vi "STM32.ADC.vi"(5 "Error":dbl, 6 "SampleRate":dbl=250000.0, 7 "Rate":dbl=1.0, 8 "Error In":errorcluster caption="错误输入", 9 "Points(X*4k)":u8=1 min=1 max=100, 10 "Channel":enum16{"Channel A", "Channel B"}(ring), 11 "VISA资源输入":refnum<visa-resource-name>) -> (0 "Error Out":errorcluster caption="错误输出", 1 "波形图":waveform(dbl)(graph), 2 "DataOut":T1)   [LabVIEW 2012, in "Lib_UEL.ATE.lvlib" / "STM32-CoreBD.lvlib"]
uses:
  STM32-CoreBD.lvlib
  <vilib>/measure/madcrms.llb/Basic Averaged DC-RMS for 1 Chan.vi
  <vilib>/measure/NI_MAPro.lvlib
panel:
  # "Version History\nV01,2014-5-04, 初始版本."
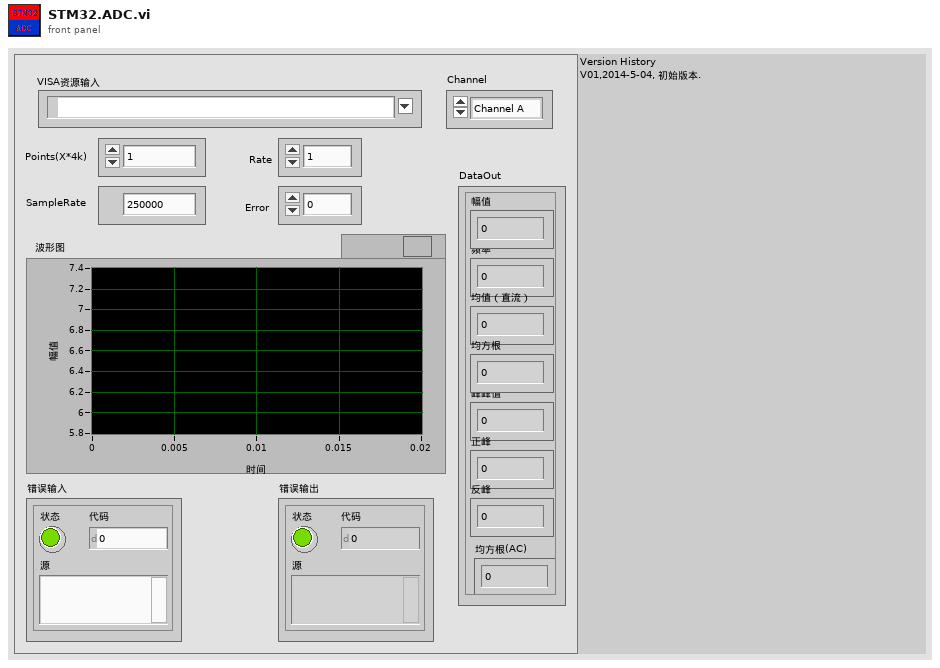
[diagram p1: front panel]
types:
  T1 = cluster{"频率":dbl, "峰峰值":dbl, "均值（直流）":dbl, "均方根":dbl, "正峰":dbl, "反峰":dbl, "幅值":dbl, "均方根(AC)":dbl}
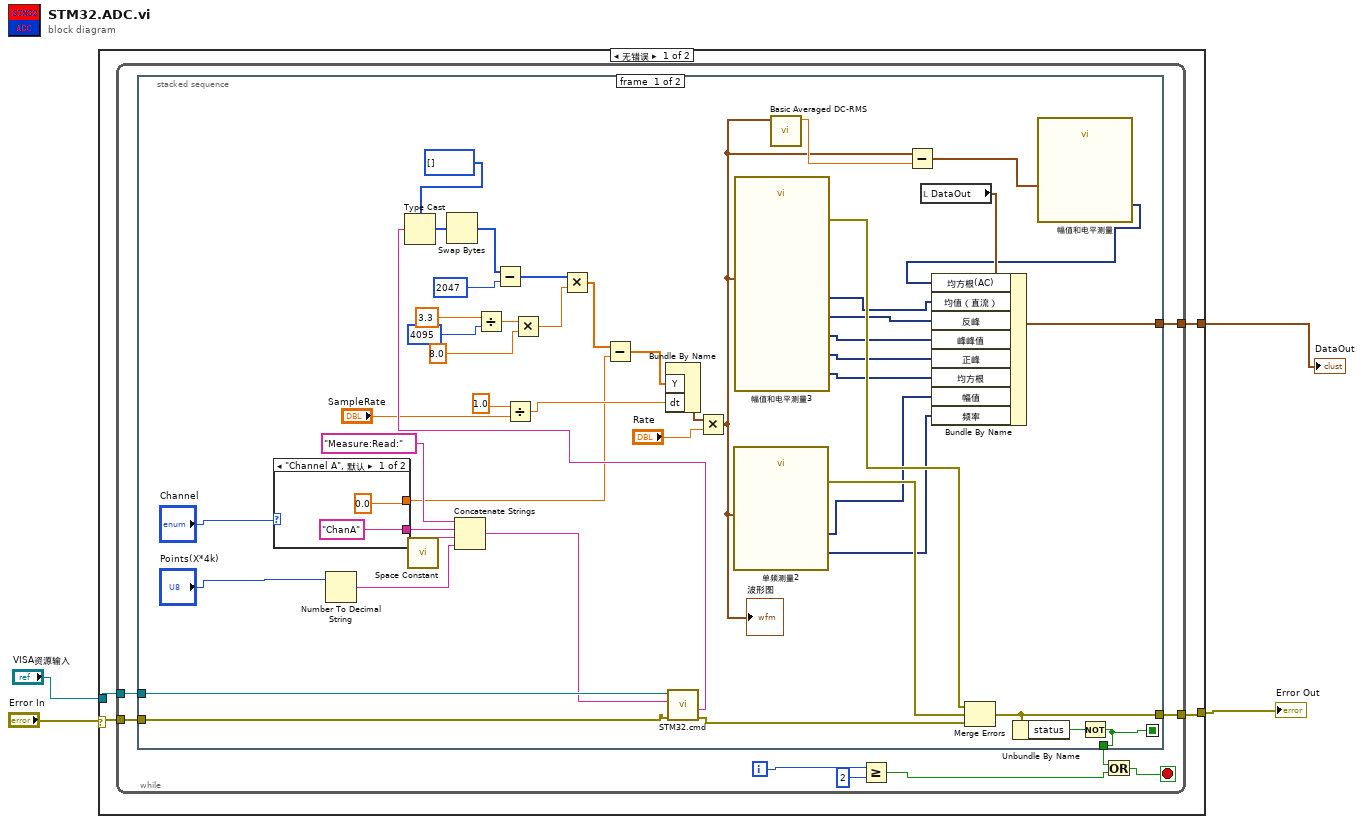
[diagram p0: block diagram]
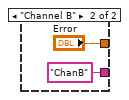
[diagram p2: hidden frame]
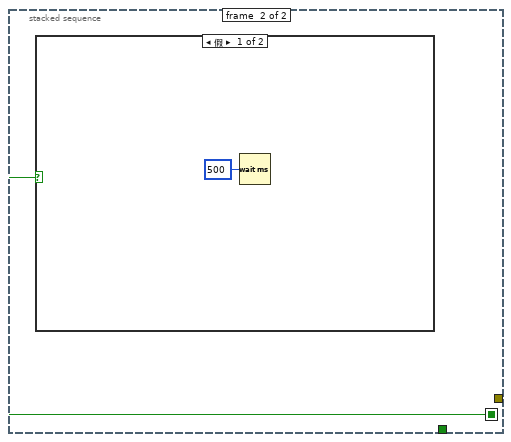
[diagram p3: hidden frame]
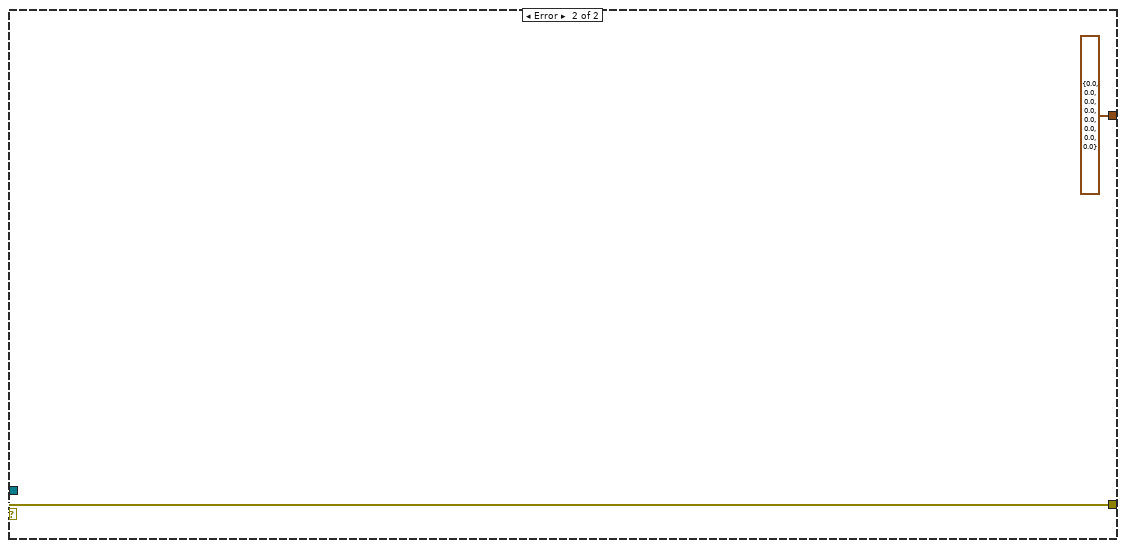
[diagram p5: hidden frame]
diagram:
  n1 = case shown="无错误" "Error In" {
    selector: "Error In" -> [w6 w72]
    tunnel: [w8 w72] -> w2
    tunnel: "VISA资源输入" -> [w7 _]
    tunnel: [w5 T1 {"频率"=0.0, "峰峰值"=0.0, "均值（直流）"=0.0, "均方根"=0.0, "正峰"=0.0, "反峰"=0.0, "幅值"=0.0, "均方根(AC)"=0.0} ("DataOut")] -> w1
    frame No Error {
      n2 = while {
        tunnel: [w14] -> w8
        tunnel: w7 -> [w17]
        tunnel: w6 -> [w16]
        tunnel: [w9] -> w5
        i -> [w12]
        stop <- w15 stop-if-true
        n3 = stacked-sequence {
          seq-local: [w34 _] -> [_ w69]
          tunnel: w17 -> [w41 _]
          tunnel: w16 -> [w40 _]
          tunnel: [w36 _] -> w14
          tunnel: [w34 _] -> w13
          tunnel: [w26 _] -> w9
          frame #0 {
            n4 = case shown="\"Channel A\", 默认" "Channel" {
              tunnel: ["ChanA" ("字符串") "ChanB" ("字符串")] -> w61
              tunnel: [0.0 "Error"] -> w27
              frame "Channel A", Default {
              }
              frame "Channel B" {
              }
            }
            n5 = Number To Decimal String(number="Points(X*4k)") -> (decimal integer string=w59:string)  [unwired: 1 in]
            n6 = call <vilib>:"Space Constant.vi"() -> ("String"=w60:string)
            n7 = Concatenate Strings("Measure:Read:" ("字符串"), w61, w60, w59) -> (w30:string)
            n8 = Divide(x=3.3 ("y"), y=4095 ("偏移量(0)")) -> (x/y=w54:dbl)
            n9 = Divide(x=1.0 ("y"), y="SampleRate") -> (x/y=w49:dbl)
            n10 = Multiply(x=w54, y=8.0) -> (x*y=w51:dbl)
            n11 = call "STM32.cmd.vi"("Error In"=w40, "命令"=w30, "VISA资源输入"=w41) -> ("Error Out"=w39:errorcluster, "附加数据"=w38:string)  [unwired: 5 in, 2 out]
            n12 = Type Cast(type=u16[] [], x=w38) -> (*(type *) &x=w57:u16[])
            n13 = Swap Bytes(anything=w57) -> (byte swapped=w56:u16[])
            n14 = Subtract(x=w56, y=2047 ("偏移量(0)")) -> (x-y=w52:i32[])
            n15 = Multiply(x=w52, y=w51) -> (x*y=w28:dbl[])
            n16 = Subtract(x=w28, y=w27) -> (x-y=w29:dbl[])
            n17 = Bundle By Name("Y"=w29, "dt"=w49) -> (w33:waveform(dbl))  [unwired: 1 in]
            n18 = Multiply(x=w33, y="Rate") -> (x*y=w24:waveform(dbl))
            "波形图" <- w24
            n19 = call "单频测量2"("Signals"=w24) -> ("error out"=w46:errorcluster, "Frequency"=w42:dynamicdata, "Amplitude"=w43:dynamicdata)  [unwired: 8 in]
            n20 = call "幅值和电平测量3"("Signals"=w24) -> ("Mean (DC)"=w20:dynamicdata, "RMS"=w21:dynamicdata, "Negative Peak"=w25:dynamicdata, "Positive Peak"=w22:dynamicdata, "Peak to Peak"=w23:dynamicdata, "error out"=w45:errorcluster)  [unwired: 9 in]
            n21 = call-poly <vilib>:"Basic Averaged DC-RMS.vi"("signal in"=w24) -> ("DC value"=w31:dbl)  [unwired: 7 in, 3 out]
            n22 = Subtract(x=w24, y=w31) -> (x-y=w19:waveform(dbl))
            n23 = local read "DataOut"() -> (w44:T1)
            n24 = Merge Errors(w45, w46, w39) -> (w36:errorcluster)
            n25 = Unbundle By Name(w36) -> ("status"=w35:bool)
            n26 = call "幅值和电平测量"("Signals"=w19) -> ("RMS"=w18:dynamicdata)  [unwired: 13 in, 1 out]
            n27 = Bundle By Name(cluster=w44, "均方根(AC)"=w18, "均值（直流）"=w20, "反峰"=w25, "峰峰值"=w23, "正峰"=w22, "均方根"=w21, "幅值"=w43, "频率"=w42) -> (w26:T1)
            n28 = Not(x=w35) -> (.not. x?=w34:bool)
          }
          frame #1 {
            n29 = case shown="假" w69 {
              frame False {
                n30 = Wait (ms)(milliseconds to wait=u32 500 ("等待时间（毫秒）")) -> ()  [unwired: 1 out]
              }
              frame True {
              }
            }
          }
        }
        n31 = Greater Or Equal?(x=w12, y=2) -> (x >= y?=w10:bool)
        n32 = Or(x=w13, y=w10) -> (x .or. y?=w15:bool)
      }
    }
    frame Error {
    }
  }
  "Error Out" <- w2
  "DataOut" <- w1
